vi "CreateMaze.vi"(8 "error in (no error)":errorcluster, 10 "MazeGameID":T1, 11 "MazeGame":refnum<class "MazeGame.lvclass">) -> (0 "error out":errorcluster, 2 "Maze":refnum<class "Maze.lvclass">, 3 "MazeGame":refnum<class "MazeGame.lvclass">)   [LabVIEW 2020, in "FactoryMethod.lvlib" / "ParameterizedFactoryMethod.lvlib" / "MazeGame.lvclass"]
uses:
  MazeGame.lvclass
  GoFcommonClasses/Maze/Maze.lvclass
  TypeDef/MazeGameID.ctl
  GoFcommonClasses/Direction.ctl
  NoParametrizedFactoryMethod/MazeGame/Private/TypeDef/RoomElement.ctl
  GoFcommonClasses/MazeSite/MazeSite.lvclass
  GoFcommonClasses/ConcreteMazeSite/Door/Door.lvclass
  E:/Francesco/GitHub/Design-Patterns-GoF_-_NI-LV/Creational/GoFcommonClasses/MazeSite/MazeSite.lvclass
  GoFcommonClasses/ConcreteMazeSite/Room/Room.lvclass
  Support/Class/ConsoleOutput.lvclass
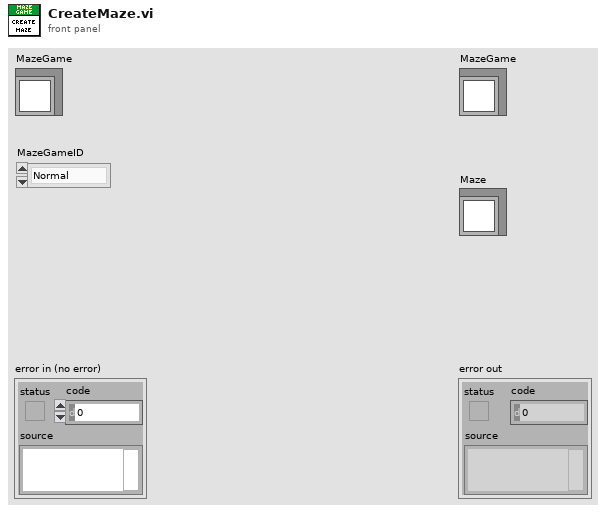
[diagram p1: front panel]
types:
  T1 = typedef "FactoryMethod.lvlib/ParameterizedFactoryMethod.lvlib/MazeGame.lvclass/MazeGameID.ctl" = enum16{"Normal", "Bombed", "Enchanted"}
  T2 = typedef "Room.lvclass/RoomElement.ctl" = cluster{"Direction":T3, "MazeSite":refnum<class "MazeSite.lvclass">}
  T3 = typedef "Direction.ctl" = enum32{"North", "South", "East", "West"}
  T4 = typedef "FactoryMethod.lvlib/ParameterizedFactoryMethod.lvlib/MazeGame.lvclass/RoomID.ctl" = enum16{"Normal", "Bombed", "Enchanted"}
  T5 = typedef "FactoryMethod.lvlib/ParameterizedFactoryMethod.lvlib/MazeGame.lvclass/WallID.ctl" = enum8{"Normal", "Bombed"}
  T6 = typedef "FactoryMethod.lvlib/ParameterizedFactoryMethod.lvlib/MazeGame.lvclass/DoorID.ctl" = enum8{"Normal", "Enchanted"}
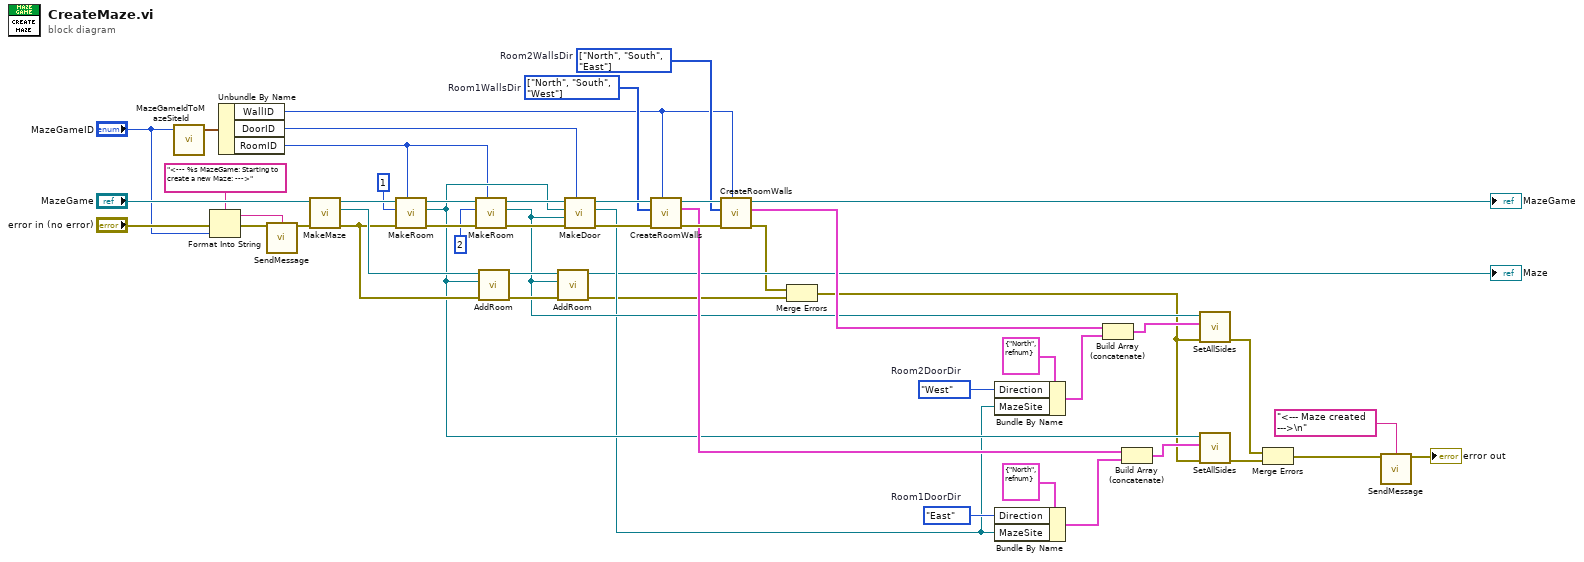
[diagram p0: block diagram]
diagram:
  w47 = Direction."West"  # Room2DoorDir
  w48 = Direction."East"  # Room1DoorDir
  w24 = T3[] [enum."North", enum."South", enum."East"] items=["North", "South", "East", "West"]  # Room2WallsDir
  w25 = T3[] [enum."North", enum."South", enum."West"] items=["North", "South", "East", "West"]  # Room1WallsDir
  n1 = call "MazeGameIdToMazeSiteId.vi"("MazeID"="MazeGameID") -> ("MazeSiteID"=w4:cluster{"RoomID":T4, "WallID":T5, "DoorID":T6})  [unwired: 4 in]
  n2 = Format Into String(format string="<--- %s MazeGame: Starting to create a new Maze: --->" ("Message"), error in="error in (no error)", "MazeGameID") -> (resulting string=w9:string, error out=w10:errorcluster)  [unwired: 1 in]
  n3 = Unbundle By Name(w4) -> ("WallID"=w1:T5, "DoorID"=w2:T6, "RoomID"=w3:T4)
  n4 = call "SendMessage.vi"("Message"=w9, "error in (no error)"=w10) -> ("error out"=w29:errorcluster)  [unwired: 13 in]
  n5 = call-dynamic "MakeMaze.vi"("error in (no error)"=w29, "MazeGame in"="MazeGame") -> ("error out"=w28:errorcluster, "Maze"=w30:refnum<class "Maze.lvclass">, "MazeGame out"=w36:refnum<class "MazeGame.lvclass">)  [unwired: 7 in]
  n6 = call-dynamic "MakeRoom.vi"("RoomID"=w3, "error in (no error)"=w28, "RoomNumber"=1, "MazeGame"=w36) -> ("error out"=w37:errorcluster, "Room"=w20:refnum<class "Room.lvclass">, "MazeGame"=w35:refnum<class "MazeGame.lvclass">)  [unwired: 5 in]
  n7 = call-dynamic "MakeRoom.vi"("RoomID"=w3, "error in (no error)"=w37, "RoomNumber"=2, "MazeGame"=w35) -> ("error out"=w32:errorcluster, "Room"=w21:refnum<class "Room.lvclass">, "MazeGame"=w31:refnum<class "MazeGame.lvclass">)  [unwired: 5 in]
  n8 = call "AddRoom.vi"("error in (no error)"=w28, "Room"=w20, "Maze in"=w30) -> ("error out"=w51:errorcluster, "Maze out"=w50:refnum<class "Maze.lvclass">)  [unwired: 7 in]
  n9 = call "AddRoom.vi"("error in (no error)"=w51, "Room"=w21, "Maze in"=w50) -> ("error out"=w17:errorcluster, "Maze out"=→"Maze":refnum<class "Maze.lvclass">)  [unwired: 7 in]
  n10 = call-dynamic "MakeDoor.vi"("DoorID"=w2, "error in (no error)"=w32, "Room 2"=w21, "Room 1"=w20, "MazeGame"=w31) -> ("error out"=w27:errorcluster, "Door"=w19:refnum<class "Door.lvclass">, "MazeGame"=w26:refnum<class "MazeGame.lvclass">)  [unwired: 4 in]
  n11 = call "CreateRoomWalls.vi"("WallID"=w1, "error in (no error)"=w27, "DirectionsList"=w25, "MazeGame"=w26) -> ("error out"=w41:errorcluster, "RoomWallsList"=w22:T2[], "MazeGame"=w40:refnum<class "MazeGame.lvclass">)  [unwired: 5 in]
  n12 = call "CreateRoomWalls.vi"("WallID"=w1, "error in (no error)"=w41, "DirectionsList"=w24, "MazeGame"=w40) -> ("error out"=w16:errorcluster, "RoomWallsList"=w23:T2[], "MazeGame"=→"MazeGame":refnum<class "MazeGame.lvclass">)  [unwired: 5 in]
  n13 = Merge Errors(w16, w17) -> (w15:errorcluster)
  n14 = Bundle By Name(cluster=T2 {"Direction"=enum."North", "MazeSite"=refnum} ("RoomElement"), "Direction"=w47, "MazeSite"=w19) -> (w44:T2)
  n15 = Bundle By Name(cluster=T2 {"Direction"=enum."North", "MazeSite"=refnum} ("RoomElement"), "Direction"=w48, "MazeSite"=w19) -> (w45:T2)
  n16 = Build Array (concatenate)(w23, w44) -> (w39:T2[])
  n17 = Build Array (concatenate)(w22, w45) -> (w38:T2[])
  n18 = call "SetAllSides.vi"("error in (no error)"=w15, "RoomSides"=w39, "Room in"=w21) -> ("error out"=w43:errorcluster)  [unwired: 7 in, 1 out]
  n19 = call "SetAllSides.vi"("error in (no error)"=w15, "RoomSides"=w38, "Room in"=w20) -> ("error out"=w42:errorcluster)  [unwired: 7 in, 1 out]
  n20 = Merge Errors(w43, w42) -> (w8:errorcluster)
  n21 = call "SendMessage.vi"("Message"="<--- Maze created --->\n" ("format string"), "error in (no error)"=w8) -> ("error out"=→"error out":errorcluster)  [unwired: 13 in]
